vi "fil_calc.vi"(6 "AI (Current Detector Output)":i16, 7 "FIFO 3":refnum<k21>="fil1.3", 8 "FIFO 2":refnum<k21>="fil1.2", 9 "FIFO 1":refnum<k21>="fil1.1", 10 "Previous Detector Correlation":i16) -> (3 "Detector Correlation Out":i16)   [LabVIEW 2015]
uses:
  <vilib>/rvi/DataTransferAndStorage/Container/Common/niFpgaContainerExecOnDevCompGetState.vi
  <vilib>/rvi/Emulation/niFpgaEmulationIsFPGAContextNoSignature.vi
  <vilib>/rvi/Emulation/niFpgaSctlEmulationGetInTimedLoop.vi
  <vilib>/rvi/errors/niFpgaSetErrorForExecOnDevCompSimple.vi
  <vilib>/rvi/eio/common/nirviEmuReportErrorAndStop.vi
  <vilib>/rvi/DataTransferAndStorage/Container/Common/niFpgaContainerGetUniqueNameForEmu.vi
  <vilib>/rvi/FIFO/Fifo_Resource/nirvififoEmulationSetSize.vi
  <vilib>/rvi/FIFO/Fifo_Resource/nirviFifoEmulationQueueMgr.vi
  <instcachedir>/0/nirviFifoEmulationQueueMgr_E5CAEC123FF24DC58D834DCA3CDAA9B5.lvgen/nirviFifoEmulationQueueMgr_E5CAEC123FF24DC58D834DCA3CDAA9B5_002.vi
  <vilib>/rvi/FIFO/Fifo_Resource/nirvififoEmulationDetermineInputValidOut.vi
  <vilib>/rvi/FIFO/Fifo_Resource/nirvififoEmulationCreateLock.vi
  <vilib>/rvi/Emulation/niFpgaProcessEmulError.vi
  <vilib>/rvi/FIFO/Fifo_Resource/nirvififoEmulationObtainLock.vi
  <vilib>/rvi/FIFO/Fifo_Resource/nirvififoEmulationReleaseLock.vi
  <vilib>/rvi/occurrence/nirviWaitOnOccurrenceBase.vi
  <vilib>/rvi/errors/nirviReportUnexpectedCaseInternalError.vi
  <vilib>/rvi/errors/nirviReportUnexpectedCaseInternalError (U32).vi
  <vilib>/Utility/error.llb/Clear Errors.vi
  <vilib>/rvi/interface/RandomDataEmulation/niFpgaRandomDataHandleErrors.vi
  <vilib>/rvi/DataTransferAndStorage/Container/XNode/niFpgaContainer.xnode
  <vilib>/rvi/FIFO/Fifo_Resource/niFpgaFifoEmulationRefIn.vi
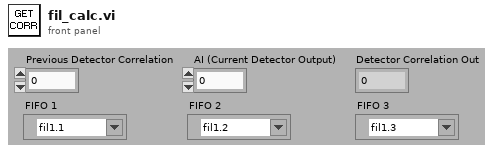
[diagram p1: front panel]
types:
  T1 = cluster{"Average Out":i32, "Next State":u16, "Detector 1 Correlation out":i32, "Detector 3 Correlation out":i32, "Velocity Count out":i32, "Detector counter out":i32, "Timeout count out":u32}
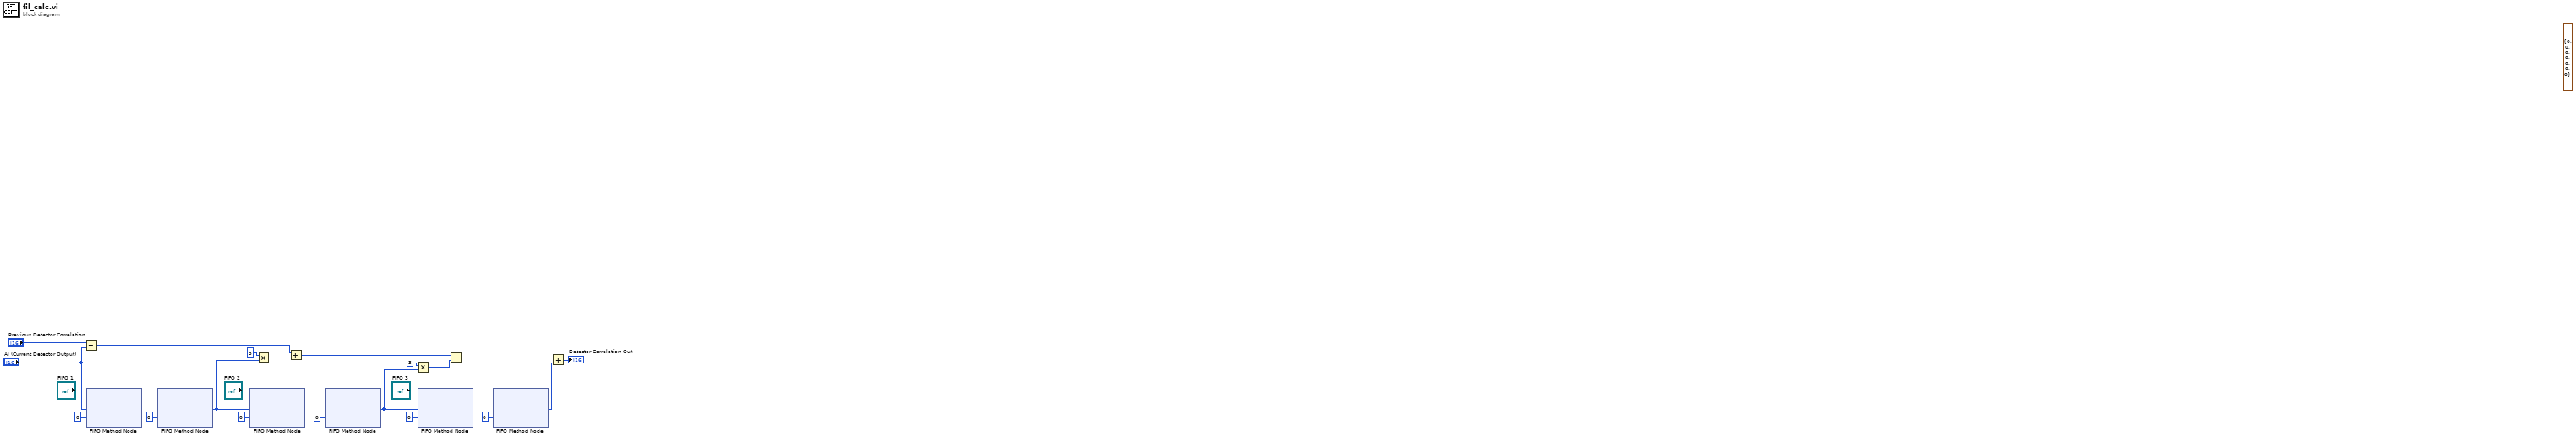
[diagram p0: block diagram]
diagram:
  (unwired) T1 {"Average Out"=0, "Next State"=0, "Detector 1 Correlation out"=0, "Detector 3 Correlation out"=0, "Velocity Count out"=0, "Detector counter out"=0, "Timeout count out"=0} ("Output Cluster")
  n1 = Subtract(x="Previous Detector Correlation", y="AI (Current Detector Output)") -> (x-y=w25:i16)
  n2 = xnode ("FIFO Method Node")("Element"="AI (Current Detector Output)", "Timeout"=0, "FIFO In"="FIFO 1") -> ("FIFO Out"=w19:refnum<k21>)  [unwired: 1 out]
  n3 = xnode ("FIFO Method Node")("Timeout"=0, "FIFO In"=w19) -> ("Element"=w11:i16)  [unwired: 2 out]
  n4 = xnode ("FIFO Method Node")("Element"=w11, "Timeout"=0, "FIFO In"="FIFO 2") -> ("FIFO Out"=w17:refnum<k21>)  [unwired: 1 out]
  n5 = Multiply(x=i16 3 ("n"), y=w11) -> (x*y=w12:i16)
  n6 = Add(x=w25, y=w12) -> (x+y=w24:i16)
  n7 = xnode ("FIFO Method Node")("Timeout"=0, "FIFO In"=w17) -> ("Element"=w6:i16)  [unwired: 2 out]
  n8 = Multiply(x=i16 3 ("n"), y=w6) -> (x*y=w4:i16)
  n9 = xnode ("FIFO Method Node")("Element"=w6, "Timeout"=0, "FIFO In"="FIFO 3") -> ("FIFO Out"=w18:refnum<k21>)  [unwired: 1 out]
  n10 = Subtract(x=w24, y=w4) -> (x-y=w23:i16)
  n11 = xnode ("FIFO Method Node")("Timeout"=0, "FIFO In"=w18) -> ("Element"=w7:i16)  [unwired: 2 out]
  n12 = Add(x=w23, y=w7) -> (x+y=→"Detector Correlation Out":i16)
